vi "Launch Async.vi"() -> ()   [LabVIEW 2021]
uses:
  Options.ctl
panel:
  in  "Launcher":i32
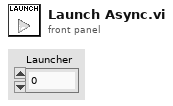
[diagram p1: front panel]
types:
  T1 = typedef "Options.ctl" = u16
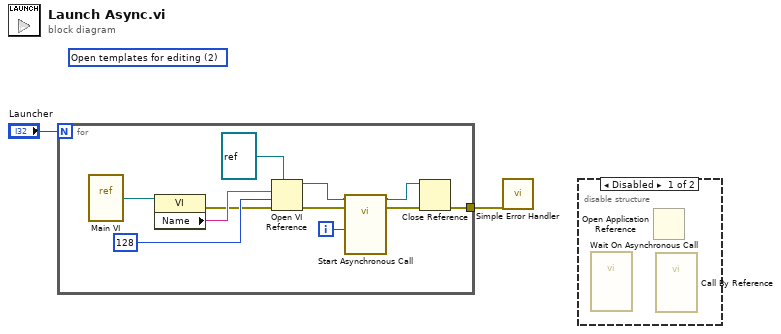
[diagram p0: block diagram]
diagram:
  (unwired) T1 2 items=["Record modifications"=1, "Open templates for editing"=2] ("Ring")
  n1 = for {
    N: "Launcher" -> [_]
    tunnel: [w6] -> w1
    i -> [w3]
    n2 = vi-ref "Main VI.vi"() -> (w13:refnum<vi>)
    n3 = property class="VI"(reference=w13) -> (error out=w10:errorcluster, "Name"=w11:string)  [unwired: 1 in, 1 out]
    n4 = Open VI Reference(type specifier VI Refnum (for type only)=refnum<vi> refnum, vi path=w11, options=128, error in (no error)=w10) -> (vi reference=w5:refnum<vi>, error out=w9:errorcluster)  [unwired: 2 in]
    n5 = call-by-ref "Start Asynchronous Call"(reference=w5, error in=w9, "Numeric"=w3) -> (reference out=w7:refnum<vi>, error out=w8:errorcluster)  [unwired: 11 in]
    n6 = Close Reference(reference=w7, error in (no error)=w8) -> (error out=w6:errorcluster)
  }
  n7 = call <vilib>:"Simple Error Handler.vi"("error in (no error)"=w1) -> ()  [unwired: 4 in, 5 out]
  n8 = disable-structure shown="Disabled" {
    frame Disabled {
      n9 = call-by-ref "Wait On Asynchronous Call"() -> ()  [unwired: 2 in, 2 out]
      n10 = Open Application Reference() -> ()  [unwired: 4 in, 2 out]
      n11 = call-by-ref "?"() -> ()  [unwired: 2 in, 2 out]
    }
    frame Enabled {
    }
  }
